vi "bic.vi"(8 "error in (no error)":errorcluster caption="entrée d'erreur (pas d'erreur)", 11 "GaussianMixture.lvclass":refnum<class "GaussianMixture.lvclass">) -> (0 "error out":errorcluster caption="sortie d'erreur", 2 "aic":dbl, 3 "GaussianMixture.lvclass 2":refnum<class "GaussianMixture.lvclass">)   [LabVIEW 2020, in "GaussianMixture.lvclass"]
doc: "Akaike information criterion for the current model on the input X."
uses:
  GaussianMixture.lvclass
  C:/Users/cipop/TDF Dropbox/2_Technologies de France/1 - Services et Etudes/PLAIY/2 - DEV/PLAIYLAB/code/Python/Python.lvclass
  C:/Users/cipop/TDF Dropbox/2_Technologies de France/1 - Services et Etudes/PLAIY/2 - DEV/PLAIYLAB/code/Model/Model.lvclass
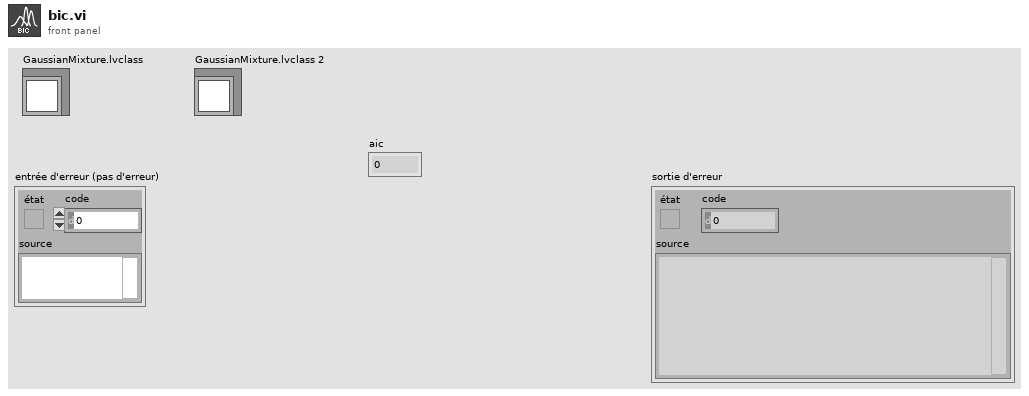
[diagram p1: front panel]
types:
  T1 = typedef "data.ctl" = cluster{"name":string, "X":dbl[][]}
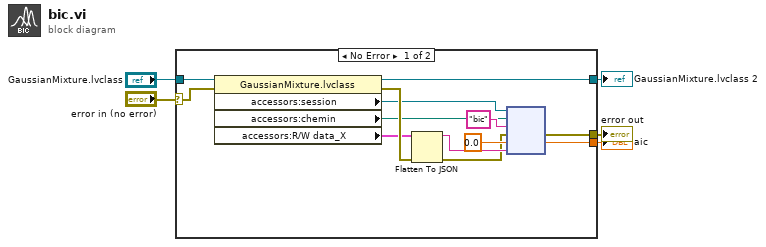
[diagram p0: block diagram]
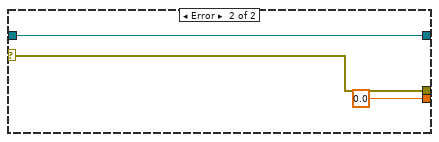
[diagram p2: hidden frame]
diagram:
  n1 = case shown="No Error" "error in (no error)" {
    selector: "error in (no error)" -> [w16 w21]
    tunnel: [w17 w21] -> w4
    tunnel: "GaussianMixture.lvclass" -> [w15 w20]
    tunnel: [w11 0.0] -> w2
    tunnel: [w7 w20] -> w1
    frame No Error {
      n2 = property class="GaussianMixture.lvclass"(reference=w15, error in=w16) -> (reference out=w7:refnum<class "GaussianMixture.lvclass">, error out=w13:errorcluster, "accessors:session"=w9:refnum<k35>, "accessors:chemin"=w8:path, "accessors:R/W data_X"=w10:T1)
      n3 = Flatten To JSON(anything=w10, error in (no error)=w13) -> (JSON string=w14:string, 11:w6:errorcluster)  [unwired: 1 in]
      n4 = node(w9, w8, "bic" ("nom de la fonction"), w6, 0.0, w14) -> (w17:errorcluster, w11:dbl)  [unwired: 1 in, 3 out]
    }
    frame Error {
    }
  }
  "error out" <- w4
  "GaussianMixture.lvclass 2" <- w1
  "aic" <- w2
